vi "Dat2Pos.vi"(0 "Draw Area Size":T2 caption="Curve Drawwing Area Size", 1 "FalseColorRatioData":T1) -> (2 "R MappedPostionInPicture":cluster{i16, i16}[](array[cluster]), 3 "G MappedPostionInPicture":cluster{i16, i16}[](array[cluster]), 4 "B MappedPostionInPicture":cluster{i16, i16}[](array[cluster]))   [LabVIEW 2016]
uses:
  <vilib>/Utility/miscctls.llb/LVBoundsTypeDef.ctl
panel:
  # "This VI is to convert ratio false color data to turn point  position in curve so can be use to draw the curve"
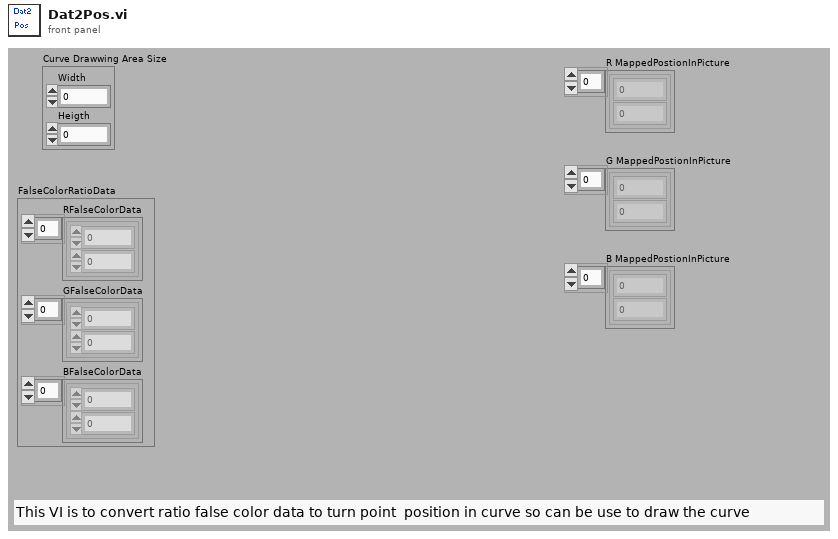
[diagram p1: front panel]
types:
  T1 = cluster{"RFalseColorData":cluster{dbl, dbl}[], "GFalseColorData":cluster{dbl, dbl}[], "BFalseColorData":cluster{dbl, dbl}[]}
  T2 = typedef "LVBoundsTypeDef.ctl" = cluster{"Width":u32, "Height":u32}
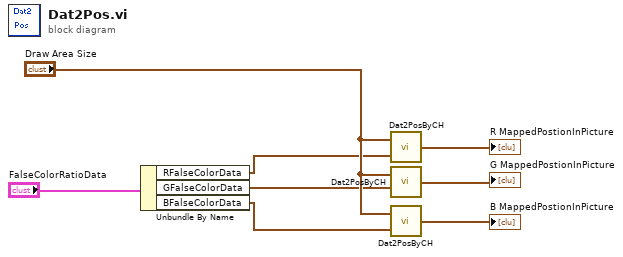
[diagram p0: block diagram]
diagram:
  n1 = Unbundle By Name("FalseColorRatioData") -> ("RFalseColorData"=w3:cluster{dbl, dbl}[], "GFalseColorData"=w2:cluster{dbl, dbl}[], "BFalseColorData"=w1:cluster{dbl, dbl}[])
  n2 = call "Dat2PosByCH.vi"("RatioClusterArray"=w3, "Draw Area Size"="Draw Area Size") -> ("MappedPostionInPicture"=→"R MappedPostionInPicture":cluster{i16, i16}[])
  n3 = call "Dat2PosByCH.vi"("RatioClusterArray"=w2, "Draw Area Size"="Draw Area Size") -> ("MappedPostionInPicture"=→"G MappedPostionInPicture":cluster{i16, i16}[])
  n4 = call "Dat2PosByCH.vi"("RatioClusterArray"=w1, "Draw Area Size"="Draw Area Size") -> ("MappedPostionInPicture"=→"B MappedPostionInPicture":cluster{i16, i16}[])
